vi "lsl library version.vi"(8 "error in (no error)":errorcluster) -> (0 "error out":errorcluster, 3 "function return":i32)   [LabVIEW 2016, in "Lab Streaming Layer.lvlib"]
doc: "extern LIBLSL_C_API int32_t lsl_library_version();"
uses:
  Lab Streaming Layer.lvlib
  liblsl-LabVIEW-master/liblsl-LabVIEW-master/lsl.dll
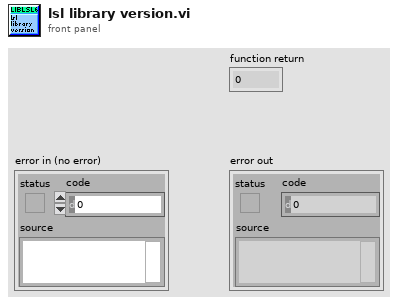
[diagram p1: front panel]
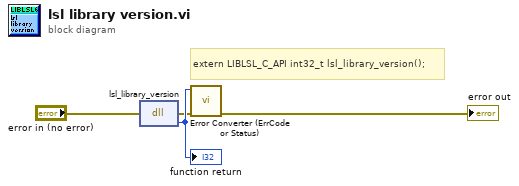
[diagram p0: block diagram]
diagram:
  # "extern LIBLSL_C_API int32_t lsl_library_version();"
  n1 = dll-call lib="E:/LabStreamingLayer/liblsl-LabVIEW-master/liblsl-LabVIEW-master/lsl.dll" fn="lsl_library_version"(error in="error in (no error)") -> (error out=w2:errorcluster, "return type"=w4:i32)  [unwired: 2 in, 1 out]
  "function return" <- w4
  n2 = call "Error Converter (ErrCode or Status).vi"("error in (no error)"=w2, "error code"=w4) -> ("error out"=→"error out":errorcluster)  [unwired: 9 in]
